vi "exists.vi"(8 "error in (no error)":errorcluster, 10 "tag":string, 11 "VGS_ComponentInfo in":refnum<class "VGS_ComponentInfo.lvclass">) -> (0 "error out":errorcluster, 2 "exists":bool, 3 "VGS_ComponentInfo out":refnum<class "VGS_ComponentInfo.lvclass">)   [LabVIEW 2022 SP3, in "LV_VGS.lvlib" / "VGS_ComponentInfo.lvclass"]
uses:
  VGS_ComponentInfo.lvclass
  VGS_ComponentInfo.lvclass/VGS_ComponentInfo.ctl
  C:/Users/Andrey/Documents/GitHub/LV_VGS/vgs_project.dll
  vgs_project.dll
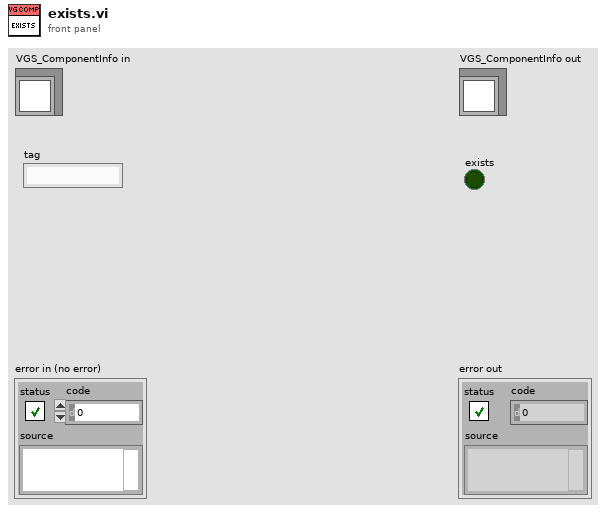
[diagram p1: front panel]
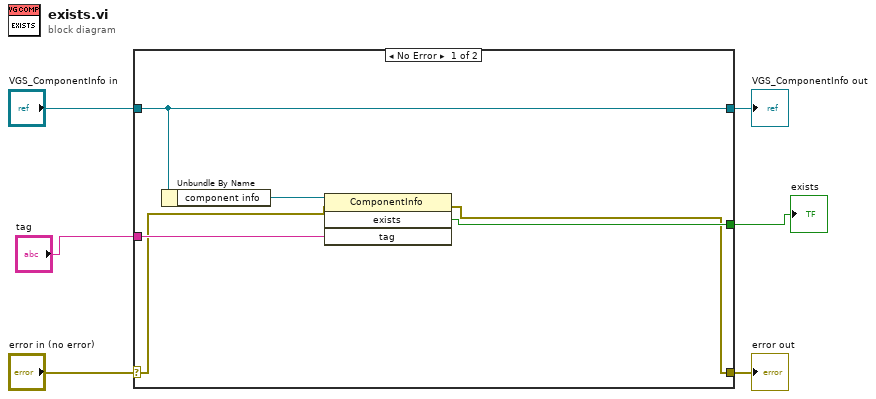
[diagram p0: block diagram]
diagram:
  n1 = case shown="No Error" "error in (no error)" {
    selector: "error in (no error)" -> [w8 w14]
    tunnel: [w7 w14] -> w5
    tunnel: [w11 w13] -> w3
    tunnel: "VGS_ComponentInfo in" -> [w11 w13]
    tunnel: [w10 _] -> w2
    tunnel: "tag" -> [w9 _]
    frame No Error {
      n2 = Unbundle By Name(w11) -> ("component info"=w12:refnum<k24>)
      n3 = invoke class="ComponentInfo" method="exists"(reference=w12, error in=w8, "tag"=w9) -> (error out=w7:errorcluster, "exists"=w10:bool)  [unwired: 1 in, 2 out]
    }
    frame Error {
    }
  }
  "error out" <- w5
  "VGS_ComponentInfo out" <- w3
  "exists" <- w2
